vi "get_serial_data.vi"(8 "error in (no error)":errorcluster, 11 "SERIAL Rsrc":string[](array[string])) -> (0 "error out":errorcluster, 1 "I/F name":string[](array[string]), 2 "COM ports":string[](array[string]), 3 "Inst ID":string[](array[string]))   [LabVIEW 2015]
uses:
  <vilib>/Instr/_visa.llb/VISA Configure Serial Port (Instr).vi
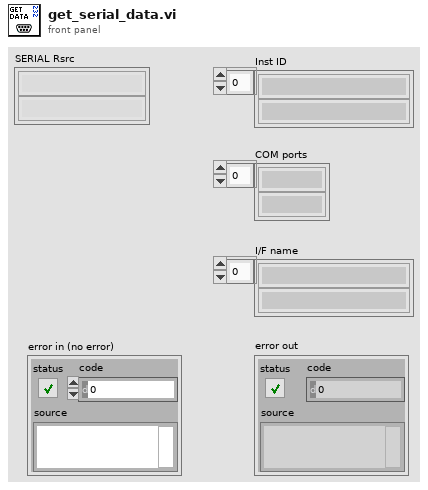
[diagram p1: front panel]
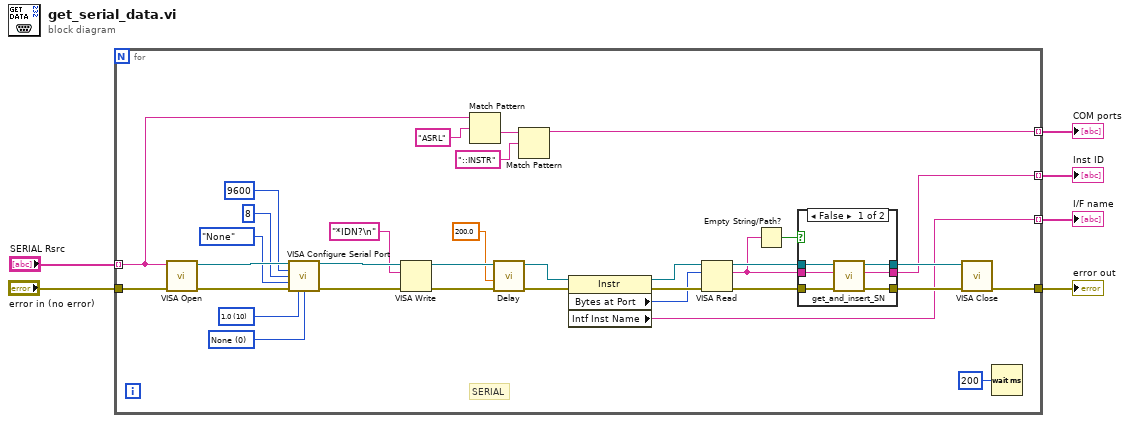
[diagram p0: block diagram]
diagram:
  n1 = for {
    tunnel: "error in (no error)" -> [w22]
    tunnel: [w17] -> w4
    tunnel: "SERIAL Rsrc" -> [w16] mode=indexing
    tunnel: [w10] -> w2 mode=indexing
    tunnel: [w18] -> w3 mode=indexing
    tunnel: [w12] -> w1 mode=indexing
    w33 = u16 0 items=["None", "XON/XOFF", "RTS/CTS", "XON/XOFF & RTS/CTS", "DTR/DSR", "XON/XOFF & DTR/DSR"] ("flow control (0:none)")
    w34 = u16 10 items=["1.0"=10, "1.5"=15, "2.0"=20] ("stop bits (10: 1 bit)")
    # "SERIAL"
    n2 = call "VISA Open.vi"("error in (no error)"=w22, "VISA resource name"=w16) -> ("error out"=w21:errorcluster, "VISA resource name out"=w38:refnum<visa-resource-name>)  [unwired: 8 in]
    n3 = call-poly "VISA Configure Serial Port"("VISA resource name"=w38, "baud rate (9600)"=u32 9600, "data bits (8)"=u16 8, "parity (0:none)"=enum16{"None", "Odd", "Even", "Mark", "Space"}."None", "error in (no error)"=w21, "stop bits (10: 1 bit)"=w34, "flow control (0:none)"=w33) -> ("VISA resource name out"=w30:refnum<visa-resource-name>, "error out"=w29:errorcluster)  [unwired: 7 in]
    n4 = VISA Write(VISA resource name=w30, write buffer="*IDN?\n", error in (no error)=w29) -> (VISA resource name out=w25:refnum<visa-resource-name>, error out=w28:errorcluster)  [unwired: 1 out]
    n5 = Match Pattern(string=w16, regular expression="ASRL") -> (after substring=w14:string)  [unwired: 1 in, 3 out]
    n6 = call "Delay.vi"("error in (no error)"=w28, "milliseconds to wait"=200.0) -> ("error out"=w31:errorcluster)  [unwired: 9 in]
    n7 = Match Pattern(string=w14, regular expression="::INSTR") -> (before substring=w12:string)  [unwired: 1 in, 3 out]
    n8 = property class="Instr"(reference=w25, error in=w31) -> (reference out=w23:refnum<visa-resource-name>, error out=w32:errorcluster, "Bytes at Port"=w9:u32, "Intf Inst Name"=w10:string)
    n9 = VISA Read(VISA resource name=w23, byte count=w9, error in (no error)=w32) -> (VISA resource name out=w19:refnum<visa-resource-name>, read buffer=w8:string, error out=w20:errorcluster)  [unwired: 1 out]
    n10 = Empty String/Path?(string/path=w8) -> (empty?=w7:bool)
    n11 = case shown="False" w7 {
      tunnel: [w45 w48] -> w39
      tunnel: w20 -> [w44 w47]
      tunnel: w19 -> [w43 w48]
      tunnel: w8 -> [w42 w46]
      tunnel: [w41 w46] -> w18
      tunnel: [w40 w47] -> w11
      frame False {
        n12 = call "get_and_insert_SN.vi"("error in (no error)"=w44, "read buffer in"=w42, "VISA Refnum in"=w43) -> ("error out"=w40:errorcluster, "read buffer out"=w41:string, "VISA Refnum out"=w45:refnum<visa-resource-name>)  [unwired: 6 in]
      }
      frame True {
      }
    }
    n13 = call "VISA Close.vi"("error in (no error)"=w11, "VISA resource name"=w39) -> ("error out"=w17:errorcluster)  [unwired: 9 in]
    n14 = Wait (ms)(milliseconds to wait=u32 200) -> ()  [unwired: 1 out]
  }
  "error out" <- w4
  "Inst ID" <- w3
  "I/F name" <- w2
  "COM ports" <- w1
